vi "isMaster.vi"(8 "error in (no error)":errorcluster, 11 "Network Master in":refnum<class "Network Master.lvclass">) -> (0 "error out":errorcluster, 2 "isMaster":bool, 3 "Network Master out":refnum<class "Network Master.lvclass">)   [LabVIEW 2012, in "Network Master.lvclass"]
uses:
  Network Master.lvclass
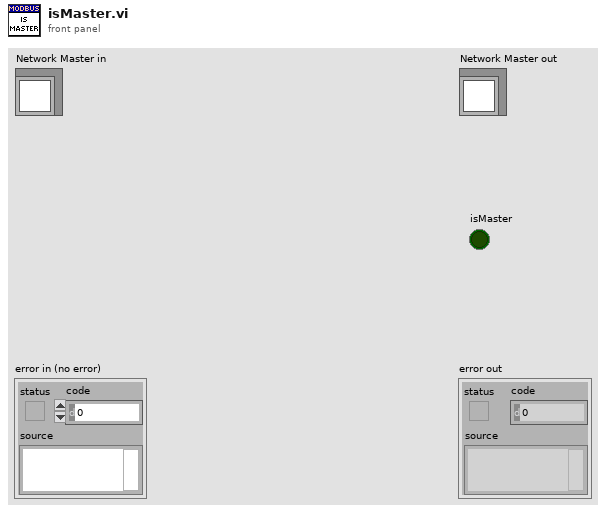
[diagram p1: front panel]
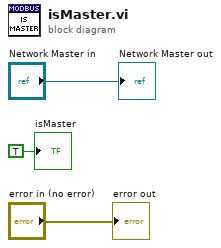
[diagram p0: block diagram]
diagram:
  "error out" <- "error in (no error)"
  "Network Master out" <- "Network Master in"
  "isMaster" <- TRUE ("isMaster")
